vi "MU Save Register.vi"(6 "values":u32[](array[numeric]), 7 "count in":u32, 8 "error in (no error)":errorcluster, 9 "address":u32, 10 "filepath":string, 11 "handle":u64) -> (0 "error out (no error)":errorcluster, 2 "count out":u32, 3 "function return":u32)   [LabVIEW 2017, in "MU_3SL_interface.lvlib"]
uses:
  MU_3SL_interface.lvlib
  lib/MU_3SL_interface.dll
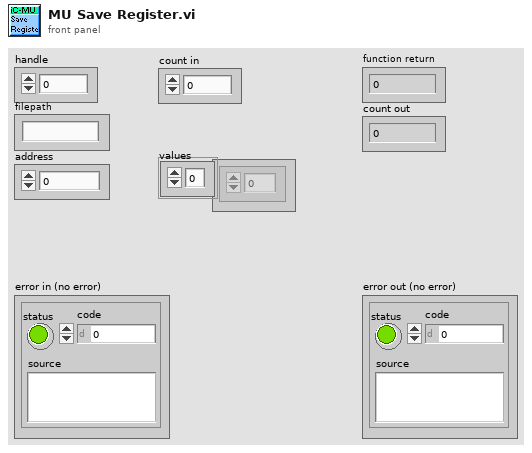
[diagram p1: front panel]
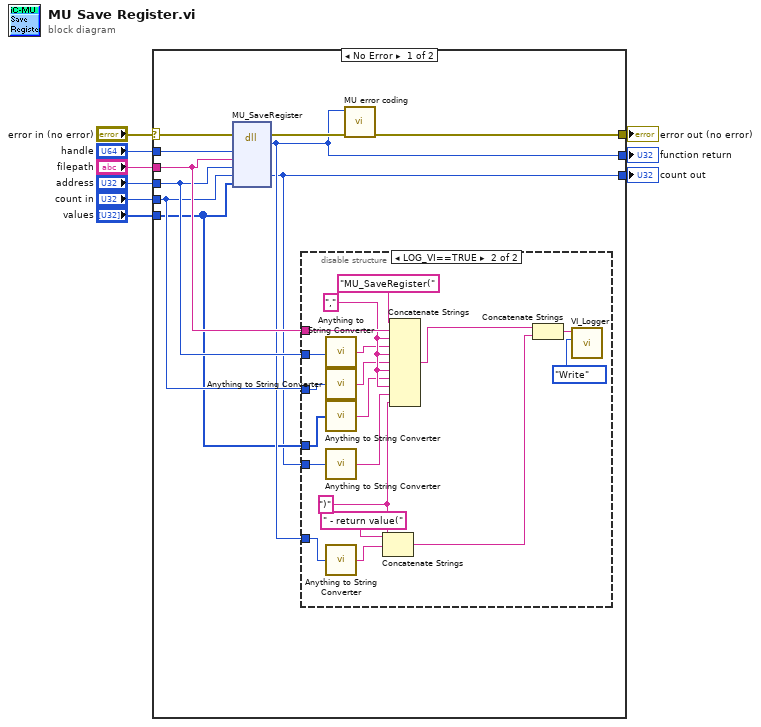
[diagram p0: block diagram]
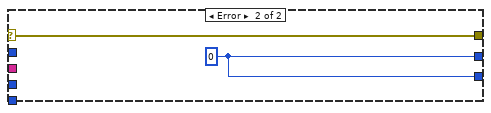
[diagram p3: hidden frame]
diagram:
  n1 = case shown="No Error" "error in (no error)" {
    selector: "error in (no error)" -> [w16 w40]
    tunnel: [w12 w39] -> w9
    tunnel: "handle" -> [w19 _]
    tunnel: "filepath" -> [w15 _]
    tunnel: "address" -> [w14 _]
    tunnel: "count in" -> [w13 _]
    tunnel: [w10 w39] -> w4
    tunnel: [w17 w40] -> w3
    tunnel: "values" -> [w11 _]
    frame No Error {
      n2 = dll-call lib="C:/Users/bes/AppData/Roaming/work/mu_9so/icsubmodules/soft_mu_3sl_master/lv_interface/lib/MU_3SL_interface**.*" fn="MU_SaveRegister"(error in=w16, "handle"=w19, "filepath"=w15, "address"=w14, "count"=w13, "values"=w11) -> (error out=w18:errorcluster, "return type"=w12:u32, "count"=w10:u32)  [unwired: 6 in, 1 out]
      n3 = disable-structure shown="LOG_VI==TRUE" {
        disable-tunnel: w12 -> [_ w22]
        disable-tunnel: w14 -> [_ w30]
        disable-tunnel: w13 -> [_ w28]
        disable-tunnel: w15 -> [_ w33]
        disable-tunnel: w11 -> [_ w26]
        disable-tunnel: w10 -> [_ w24]
        frame condition #0 {
        }
        frame condition #1 (active) {
          w32 = ")" ("string")
          w31 = "," ("string")
          n4 = call "Anything to String Converter.vi"("anything"=w30) -> ("String"=w29:string)
          n5 = call "Anything to String Converter.vi"("anything"=w28) -> ("String"=w27:string)
          n6 = call "Anything to String Converter.vi"("anything"=w26) -> ("String"=w25:string)
          n7 = call "Anything to String Converter.vi"("anything"=w24) -> ("String"=w23:string)
          n8 = call "Anything to String Converter.vi"("anything"=w22) -> ("String"=w21:string)
          n9 = Concatenate Strings(" - return value(" ("string"), w21, w32) -> (w36:string)
          n10 = Concatenate Strings("MU_SaveRegister(" ("Info in"), w33, w31, w29, w31, w27, w31, w25, w31, w23, w32) -> (w20:string)
          n11 = Concatenate Strings(w20, w36) -> (w35:string)
          n12 = call "VI_Logger.vi"("Action (Read)"=enum16{"Write", "Read"}."Write", "Info in"=w35) -> ()  [unwired: 8 in, 2 out]
        }
      }
      n13 = call "MU error coding.vi"("error in (no error)"=w18, "function return in"=w12) -> ("error out"=w17:errorcluster)  [unwired: 9 in]
    }
    frame Error {
      w39 = u32 0 ("return type")
    }
  }
  "function return" <- w9
  "count out" <- w4
  "error out (no error)" <- w3
